vi "EminemExecuteLogic.vi"(9 "Feed_Vel_RPM":dbl, 10 "Shooter_Bottom_Vel_RPM":dbl, 11 "Shooter_Top_Vel_RPM":dbl) -> (0 "Box states":T1=enum."13-AmpDone", 1 "Shooter_Feed_Motor_Out":dbl, 2 "Shooter_Bottom_Motor_Out":dbl, 3 "Shooter_Top_Motor_Out":dbl)   [LabVIEW 2023]
uses:
  EminemStatesEnum.ctl
  <vilib>/Rock Robotics/WPI/ThirdParty/JAS_Junk/TrajLib/TypeDef/PID_ERROR_TOLERANCE.ctl
  <vilib>/Rock Robotics/WPI/ThirdParty/JAS_Junk/TrajLib/LinearFilter_ResetToValue.vi
  <vilib>/Rock Robotics/WPI/ThirdParty/JAS_Junk/TrajLib/LinearFilter_Calculate.vi
  <vilib>/Rock Robotics/WPI/ThirdParty/JAS_Junk/TrajLib/VI/BoolCmd_Recv_Internal.vi
  <vilib>/Rock Robotics/WPI/ThirdParty/JAS_Junk/TrajLib/Timer_New.vi
  Intake/IntakeGetHaveNote.vi
  <vilib>/Rock Robotics/WPI/ThirdParty/JAS_Junk/TrajLib/SlewRateLimiter_New.vi
  <vilib>/Rock Robotics/WPI/ThirdParty/JAS_Junk/TrajLib/SlewRateLimiter_Reset.vi
  <vilib>/Rock Robotics/WPI/ThirdParty/JAS_Junk/TrajLib/SlewRateLimiter_Calculate.vi
  <vilib>/Rock Robotics/WPI/ThirdParty/JAS_Junk/TrajLib/SlewRateLimiter_SetRate.vi
  <vilib>/Rock Robotics/WPI/ThirdParty/JAS_Junk/TrajLib/SimpleMotorFF_Calculate.vi
  <vilib>/Rock Robotics/WPI/ThirdParty/JAS_Junk/TrajLib/PIDController_AtSetpoint.vi
  <vilib>/Rock Robotics/WPI/ThirdParty/JAS_Junk/TrajLib/PIDController_SetPIDF.vi
  <vilib>/Rock Robotics/WPI/ThirdParty/JAS_Junk/TrajLib/PIDController_SetDerivativeFilter.vi
  <vilib>/Rock Robotics/WPI/ThirdParty/JAS_Junk/TrajLib/PIDController_SetIntegratorRange.vi
  <vilib>/Rock Robotics/WPI/ThirdParty/JAS_Junk/TrajLib/PIDController_SetTolerancePandV.vi
  <vilib>/Rock Robotics/WPI/ThirdParty/JAS_Junk/TrajLib/PIDController_DisableContinousInput.vi
  <vilib>/Rock Robotics/WPI/ThirdParty/JAS_Junk/TrajLib/PIDController_EnableContinousInput.vi
  <vilib>/Rock Robotics/WPI/ThirdParty/JAS_Junk/TrajLib/PIDController_Reset.vi
  <vilib>/Rock Robotics/WPI/ThirdParty/JAS_Junk/TrajLib/PIDController_New.vi
  <vilib>/Rock Robotics/WPI/ThirdParty/JAS_Junk/TrajLib/PIDController_SetOutputLimits.vi
  <vilib>/Rock Robotics/WPI/ThirdParty/JAS_Junk/TrajLib/VI/PIDController_SetIntegratorZone.vi
  <vilib>/Rock Robotics/WPI/ThirdParty/JAS_Junk/TrajLib/VI/BoolCmd_ObtainQueue.vi
  <vilib>/Rock Robotics/WPI/ThirdParty/JAS_Junk/TrajLib/Util_GetTime.vi
  <vilib>/Rock Robotics/WPI/ThirdParty/JAS_Junk/TrajLib/PIDController_NewPeriod.vi
  <vilib>/Rock Robotics/WPI/ThirdParty/JAS_Junk/TrajLib/VI/Util_GetTime_U32.vi
  <vilib>/Rock Robotics/SystemInterfaces/NetworkCommunication/NetComm_UsageReport_report.vi
  EminemGlobals.vi
  <vilib>/Utility/semaphor.llb/Obtain Semaphore Reference.vi
  <vilib>/Rock Robotics/WPI/ThirdParty/JAS_Junk/TrajLib/Timer_Reset.vi
  Intake/IntakeGlobal.vi
  Intake/IntakeCmdCancelALWAYS.vi
  <vilib>/Rock Robotics/WPI/ThirdParty/JAS_Junk/TrajLib/VI/Timer_Restart.vi
  <vilib>/Rock Robotics/WPI/ThirdParty/JAS_Junk/TrajLib/Timer_HasPeriodPassedOnce.vi
  Intake/IntakeCmdFeedToShootALWAYS.vi
  <vilib>/Rock Robotics/WPI/ThirdParty/JAS_Junk/TrajLib/VI/Util_GetTime_U64.vi
  <vilib>/Rock Robotics/WPI/ThirdParty/JAS_Junk/TrajLib/LinearFilter_MovingAverage.vi
  <vilib>/Rock Robotics/WPI/ThirdParty/JAS_Junk/TrajLib/LinearFilter_LowPassBW1.vi
  <vilib>/Rock Robotics/WPI/ThirdParty/JAS_Junk/TrajLib/LinearFilter_LowPassBW2.vi
  <vilib>/Rock Robotics/WPI/ThirdParty/JAS_Junk/TrajLib/LinearFilter_HighPassBW1.vi
  <vilib>/Rock Robotics/WPI/ThirdParty/JAS_Junk/TrajLib/LinearFilter_HighPassBW2.vi
  <vilib>/Rock Robotics/WPI/ThirdParty/JAS_Junk/TrajLib/Globals/Util_LibraryGlobals.vi
  <vilib>/Rock Robotics/WPI/ThirdParty/JAS_Junk/TrajLib/PIDController_AdvCalculate_FF_Sp_Pv.vi
  <vilib>/Rock Robotics/WPI/ThirdParty/JAS_Junk/TrajLib/Trajectory_Library.lvlib
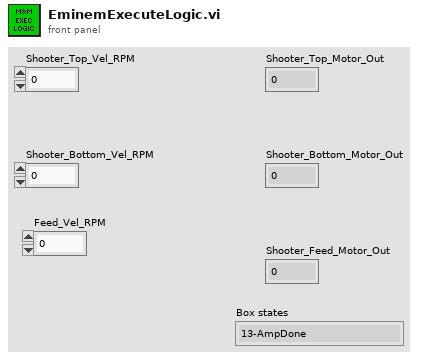
[diagram p1: front panel]
types:
  T1 = typedef "EminemStatesEnum.ctl" = enum16{"0-Init", "1-WaitForCmd", "2-Cancel", "3-ShootStart", "4-ShootRev", "5-RevUpStart", "6-ShootStartFeed&Timer", "7-ShootTimerOrSensorDone", "8-ShootDone", "9-AmpStart", "10-AmpUpToSpd?", "11-AmpStartFeed&Timer", "12-AmpTimerOrSensorDone", "13-AmpDone", "14-RevUpGetCmd"}
  T2 = enum16{"Moving Average", "Low Pass 1st Order Butterworth", "Low Pass 2nd Order Butterworth", "High Pass 1st Order Butterworth", "High Pass 2nd Order Butterworth"}
  T3 = typedef "Trajectory_Library.lvlib/PID_ERROR_TOLERANCE.ctl" = cluster{"PositionTolerance":dbl, "VelocityTolerance":dbl}
  T4 = typedef "Trajectory_Library.lvlib/SIMPLE_MOTOR_FF.ctl" = cluster{"Ks":dbl, "Kv":dbl, "Ka":dbl, "KnInv":dbl}
  T5 = typedef "Trajectory_Library.lvlib/PID_ADV_TUNING.ctl" = cluster{"Kf":dbl, "Kp":dbl, "Ki":dbl, "Kd":dbl, "MaximumIntegral":dbl, "MinimumIntegral":dbl, "Filter Derivative":bool, "IntegralZone":dbl}
  T6 = typedef "Trajectory_Library.lvlib/PID_ADV_LIMITS.ctl" = cluster{"MaxInput":dbl, "MinInput":dbl, "Continuous":bool, "MaxOutput":dbl, "MinOutput":dbl}
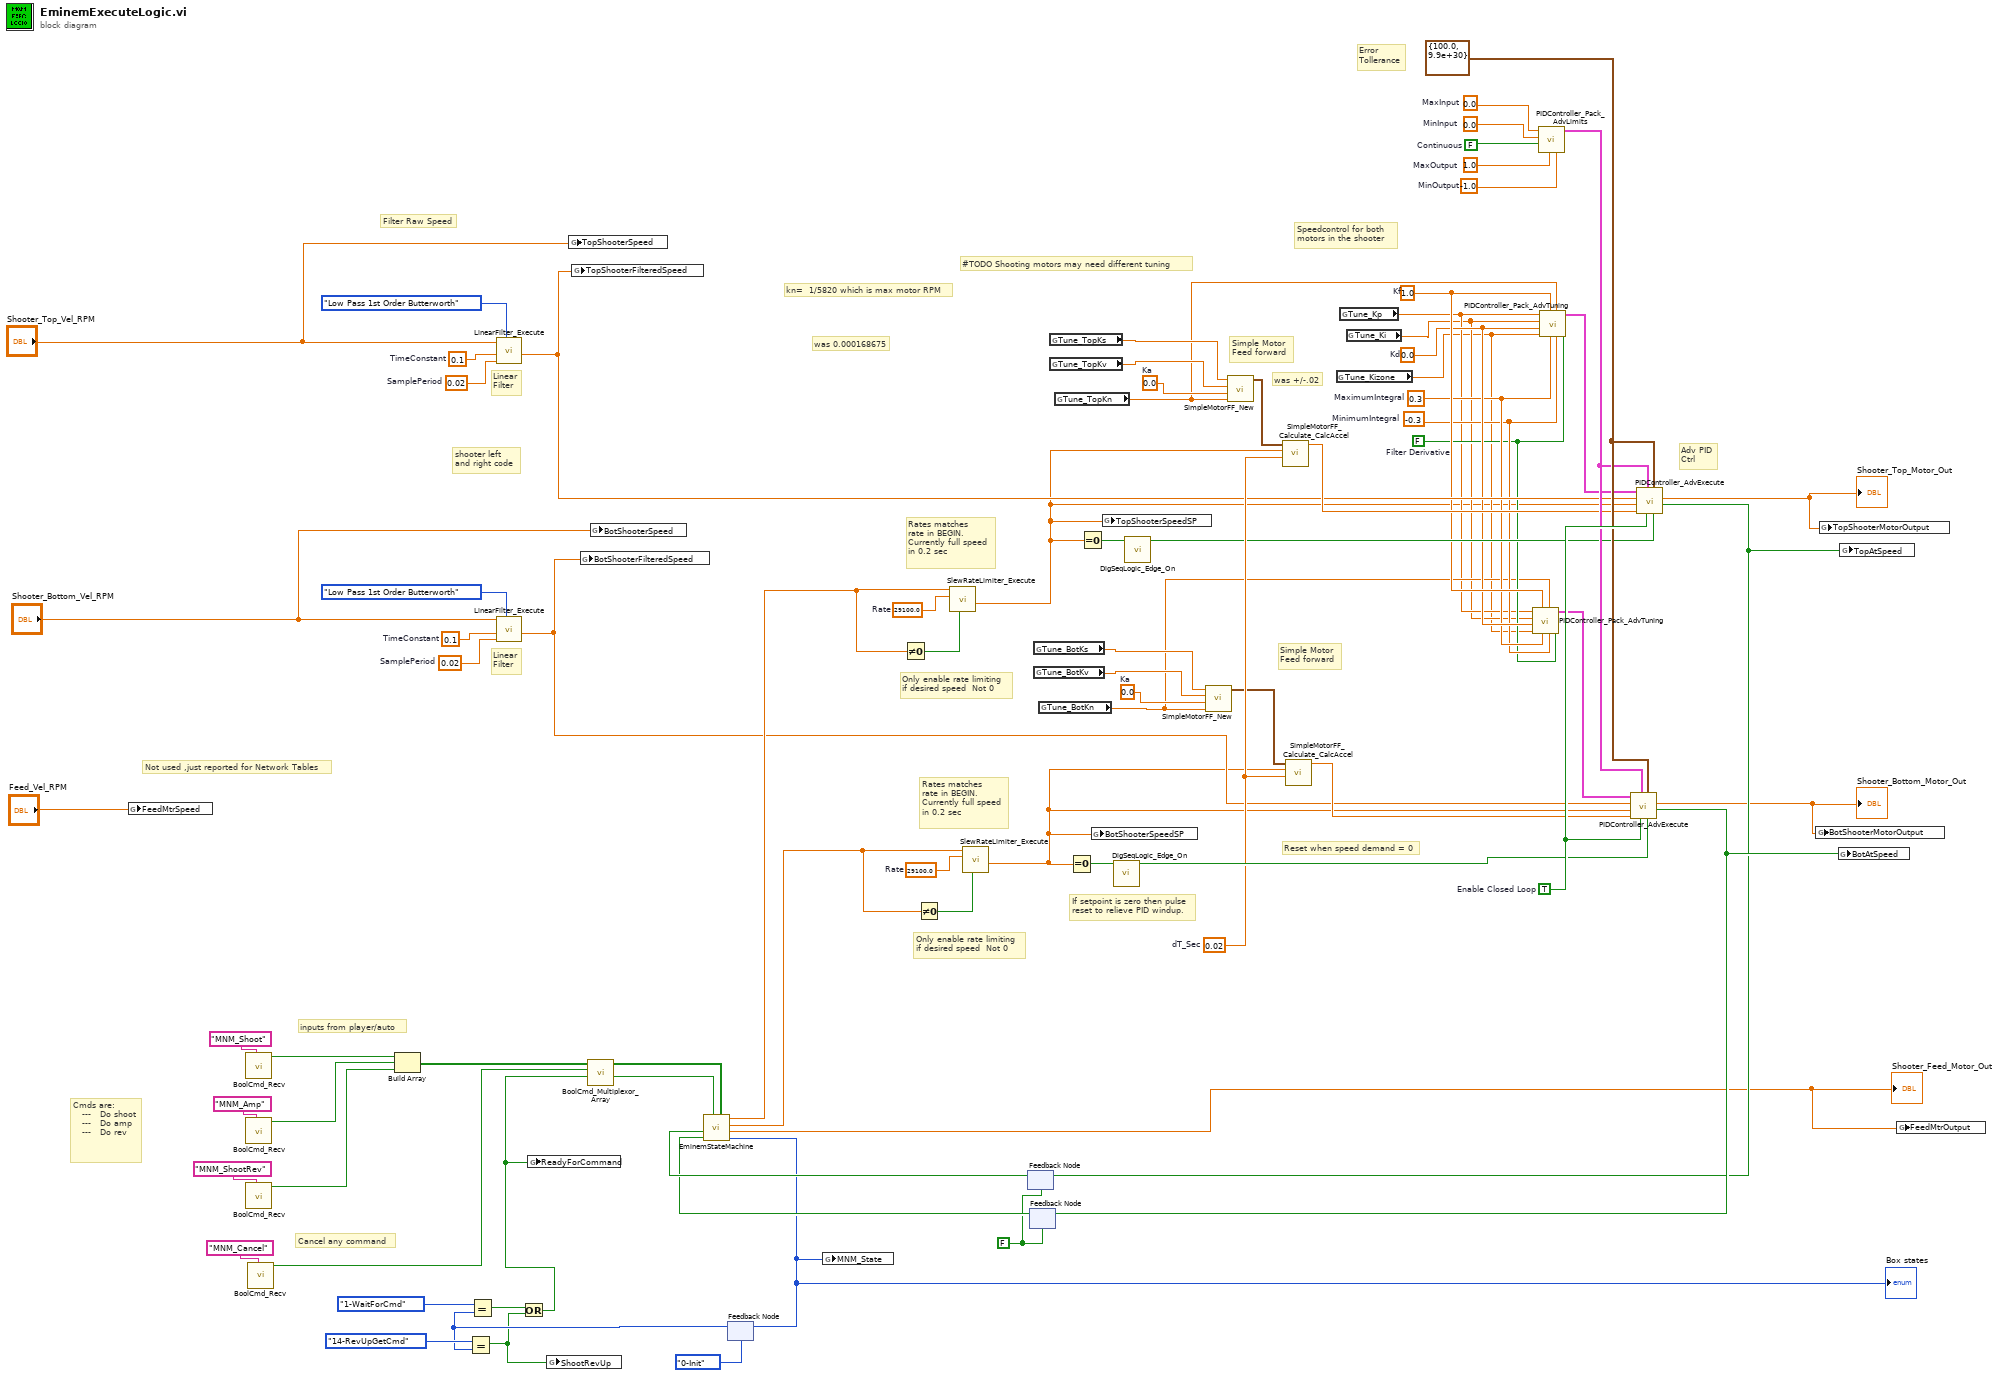
[diagram p0: block diagram]
diagram:
  w19 = 0.0  # Ka
  w26 = FALSE ("AtSetpoint")
  w42 = 29100.0  # Rate
  w79 = 29100.0  # Rate
  w74 = 0.02  # SamplePeriod
  w75 = 0.1  # TimeConstant
  w71 = 0.02  # SamplePeriod
  w72 = 0.1  # TimeConstant
  w81 = TRUE  # Enable Closed Loop
  w69 = T3 {"PositionTolerance"=100.0, "VelocityTolerance"=9.9e+30} ("PID Error Tolerance")
  w64 = 0.0  # Ka
  w15 = 0.0  # Kd
  w16 = 1.0  # Kf
  w14 = 0.3  # MaximumIntegral
  w13 = -0.3  # MinimumIntegral
  w12 = FALSE  # Filter Derivative
  w60 = 0.0  # MinInput
  w61 = FALSE  # Continuous
  w62 = 1.0  # MaxOutput
  w63 = -1.0  # MinOutput
  w59 = 0.0  # MaxInput
  w65 = 0.02  # dT_Sec
  # "Simple Motor\nFeed forward"
  # "was 0.000168675"
  # "#TODO Shooting motors may need different tuning"
  # "Not used ,just reported for Network Tables"
  # "Cmds are:\n   ---   Do shoot\n   ---   Do amp\n   ---   Do rev"
  # "Error \nTollerance"
  # "Filter Raw Speed"
  # "Rates matches\nrate in BEGIN.  \nCurrently full speed\nin 0.2 sec"
  # "Only enable rate limiting\nif desired speed  Not 0"
  # "Reset when speed demand = 0"
  # "was +/-.02"
  # "If setpoint is zero then pulse\nreset to relieve PID windup."
  # "Rates matches\nrate in BEGIN.  \nCurrently full speed\nin 0.2 sec"
  # "Only enable rate limiting\nif desired speed  Not 0"
  # "inputs from player/auto"
  # "Linear\nFilter"
  # "Linear\nFilter"
  # "Speedcontrol for both \nmotors in the shooter"
  # "Simple Motor\nFeed forward"
  # "Adv PID\nCtrl"
  # "Cancel any command"
  # "kn=  1/5820 which is max motor RPM"
  # "shooter left \nand right code"
  n1 = global write "EminemGlobals.vi" "FeedMtrSpeed"("Feed_Vel_RPM") -> ()
  n2 = call <vilib>:"BoolCmd_Recv.vi"("Command Name"="MNM_Shoot") -> ("New Request"=w52:bool)  [unwired: 9 in, 1 out]
  n3 = call <vilib>:"BoolCmd_Recv.vi"("Command Name"="MNM_Amp") -> ("New Request"=w51:bool)  [unwired: 9 in, 1 out]
  n4 = call <vilib>:"BoolCmd_Recv.vi"("Command Name"="MNM_ShootRev") -> ("New Request"=w49:bool)  [unwired: 9 in, 1 out]
  n5 = call <vilib>:"BoolCmd_Recv.vi"("Command Name"="MNM_Cancel") -> ("New Request"=w54:bool)  [unwired: 9 in, 1 out]
  n6 = Build Array(w52, w51, w49) -> (w53:bool[])
  n7 = call <vilib>:"LinearFilter_Execute.vi"("Filter Type"=T2."Low Pass 1st Order Butterworth", "SamplePeriod"=w74, "TimeConstant"=w75, "Input"="Shooter_Top_Vel_RPM") -> ("Output"=w28:dbl)  [unwired: 6 in, 1 out]
  n8 = call <vilib>:"LinearFilter_Execute.vi"("Filter Type"=T2."Low Pass 1st Order Butterworth", "SamplePeriod"=w71, "TimeConstant"=w72, "Input"="Shooter_Bottom_Vel_RPM") -> ("Output"=w30:dbl)  [unwired: 6 in, 1 out]
  n9 = global write "EminemGlobals.vi" "TopShooterSpeed"("Shooter_Top_Vel_RPM") -> ()
  n10 = global write "EminemGlobals.vi" "TopShooterFilteredSpeed"(w28) -> ()
  n11 = global write "EminemGlobals.vi" "BotShooterFilteredSpeed"(w30) -> ()
  n12 = global write "EminemGlobals.vi" "BotShooterSpeed"("Shooter_Bottom_Vel_RPM") -> ()
  n13 = feedback #1(EminemStatesEnum."0-Init" ("Box states")) -> (w23:T1)
  n14 = Equal?(x=EminemStatesEnum."14-RevUpGetCmd" ("Box states"), y=w23) -> (x = y?=w20:bool)
  n15 = Equal?(x=EminemStatesEnum."1-WaitForCmd" ("Box states"), y=w23) -> (x = y?=w22:bool)
  n16 = Or(x=w22, y=w20) -> (x .or. y?=w21:bool)
  n17 = global write "EminemGlobals.vi" "ReadyForCommand"(w21) -> ()
  n18 = global write "EminemGlobals.vi" "ShootRevUp"(w20) -> ()
  n19 = call <vilib>:"BoolCmd_Multiplexor_Array.vi"("Ready"=w21, "Command Cancel"=w54, "Commands"=w53) -> ("Do Cancel"=w45:bool, "Do Command"=w46:bool[])  [unwired: 7 in]
  n20 = feedback #2(w26) -> (w41:bool)
  n21 = feedback #3(w26) -> (w40:bool)
  n22 = call "EminemStateMachine.vi"("EminemCommand"=w46, "EminemCancel"=w45, "LowerShoot_At_Speed"=w40, "UpperShoot_At_Speed"=w41) -> ("Box states"=w37:T1, "AmpAndFeed-MotorDmd"=w32:dbl, "LowerShooter-RPM_Dmd"=w39:dbl, "UpperShooterAndAmp-RPM_Dmd"=w38:dbl)  [unwired: 4 in]
  "Shooter_Feed_Motor_Out" <- w32
  "Box states" <- w37
  n23 = feedback-in #1(w37) -> ()
  n24 = global write "EminemGlobals.vi" "MNM_State"(w37) -> ()
  n25 = Not Equal To 0?(x=w38) -> (x != 0?=w43:bool)
  n26 = Not Equal To 0?(x=w39) -> (x != 0?=w80:bool)
  n27 = call <vilib>:"SlewRateLimiter_Execute.vi"("Enable"=w43, "PositiveRate"=w42, "Input"=w38) -> ("Output"=w2:dbl)  [unwired: 7 in, 1 out]
  n28 = call <vilib>:"SlewRateLimiter_Execute.vi"("Enable"=w80, "PositiveRate"=w79, "Input"=w39) -> ("Output"=w1:dbl)  [unwired: 7 in, 1 out]
  n29 = global read "EminemGlobals.vi" "Tune_BotKs"() -> (w8:dbl)
  n30 = global read "EminemGlobals.vi" "Tune_BotKv"() -> (w7:dbl)
  n31 = global read "EminemGlobals.vi" "Tune_BotKn"() -> (w6:dbl)
  n32 = global read "EminemGlobals.vi" "Tune_TopKs"() -> (w11:dbl)
  n33 = global read "EminemGlobals.vi" "Tune_TopKv"() -> (w10:dbl)
  n34 = global read "EminemGlobals.vi" "Tune_TopKn"() -> (w9:dbl)
  n35 = Equal To 0?(x=w1) -> (x = 0?=w77:bool)
  n36 = Equal To 0?(x=w2) -> (x = 0?=w48:bool)
  n37 = global write "EminemGlobals.vi" "BotShooterSpeedSP"(w1) -> ()
  n38 = global write "EminemGlobals.vi" "TopShooterSpeedSP"(w2) -> ()
  n39 = call <vilib>:"DigSeqLogic_Edge_On.vi"("Input"=w77) -> ("On Edge"=w78:bool)  [unwired: 10 in]
  n40 = call <vilib>:"DigSeqLogic_Edge_On.vi"("Input"=w48) -> ("On Edge"=w47:bool)  [unwired: 10 in]
  n41 = call <vilib>:"SimpleMotorFF_New.vi"("Kn"=w6, "Ka"=w19, "Kv"=w7, "Ks"=w8) -> ("SIMPLE_MOTOR_FF"=w18:T4)  [unwired: 7 in]
  n42 = call <vilib>:"SimpleMotorFF_New.vi"("Kn"=w9, "Ka"=w64, "Kv"=w10, "Ks"=w11) -> ("SIMPLE_MOTOR_FF"=w66:T4)  [unwired: 7 in]
  n43 = call <vilib>:"SimpleMotorFF_Calculate_CalcAccel.vi"("dT_Sec"=w65, "VelSp"=w2, "SIMPLE_MOTOR_FF"=w66) -> ("FeedForward"=w58:dbl)  [unwired: 8 in]
  n44 = call <vilib>:"SimpleMotorFF_Calculate_CalcAccel.vi"("dT_Sec"=w65, "VelSp"=w1, "SIMPLE_MOTOR_FF"=w18) -> ("FeedForward"=w70:dbl)  [unwired: 8 in]
  n45 = global read "EminemGlobals.vi" "Tune_Kizone"() -> (w3:dbl)
  n46 = global read "EminemGlobals.vi" "Tune_Kp"() -> (w5:dbl)
  n47 = global read "EminemGlobals.vi" "Tune_Ki"() -> (w4:dbl)
  n48 = call <vilib>:"PIDController_Pack_AdvTuning.vi"("Filter Derivative"=w12, "MinimumIntegral"=w13, "Kn"=w6, "MaximumIntegral"=w14, "Kf"=w16, "IntegralZone"=w3, "Kd"=w15, "Ki"=w4, "Kp"=w5) -> ("Adv PID Tuning"=w17:T5)  [unwired: 2 in]
  n49 = call <vilib>:"PIDController_Pack_AdvLimits.vi"("MinOutput"=w63, "MaxOutput"=w62, "Continuous"=w61, "MinInput"=w60, "MaxInput"=w59) -> ("Adv PID Limits"=w68:T6)  [unwired: 6 in]
  n50 = call <vilib>:"PIDController_Pack_AdvTuning.vi"("Filter Derivative"=w12, "MinimumIntegral"=w13, "Kn"=w9, "MaximumIntegral"=w14, "Kf"=w16, "IntegralZone"=w3, "Kd"=w15, "Ki"=w4, "Kp"=w5) -> ("Adv PID Tuning"=w67:T5)  [unwired: 2 in]
  n51 = call <vilib>:"PIDController_AdvExecute.vi"("Reset"=w78, "PID Error Tolerance"=w69, "Auto"=w81, "Adv PID Limits"=w68, "FF-FeedForward"=w70, "SP-SetPoint"=w1, "PV-Measurement"=w30, "Adv PID Tuning"=w17) -> ("AtSetpoint"=w36:bool, "CO-ControlOutput"=w33:dbl)  [unwired: 1 in, 1 out]
  "Shooter_Bottom_Motor_Out" <- w33
  n52 = feedback-in #3(w36) -> ()
  n53 = call <vilib>:"PIDController_AdvExecute.vi"("Reset"=w47, "PID Error Tolerance"=w69, "Auto"=w81, "Adv PID Limits"=w68, "FF-FeedForward"=w58, "SP-SetPoint"=w2, "PV-Measurement"=w28, "Adv PID Tuning"=w67) -> ("AtSetpoint"=w35:bool, "CO-ControlOutput"=w34:dbl)  [unwired: 1 in, 1 out]
  "Shooter_Top_Motor_Out" <- w34
  n54 = feedback-in #2(w35) -> ()
  n55 = global write "EminemGlobals.vi" "BotShooterMotorOutput"(w33) -> ()
  n56 = global write "EminemGlobals.vi" "TopShooterMotorOutput"(w34) -> ()
  n57 = global write "EminemGlobals.vi" "BotAtSpeed"(w36) -> ()
  n58 = global write "EminemGlobals.vi" "TopAtSpeed"(w35) -> ()
  n59 = global write "EminemGlobals.vi" "FeedMtrOutput"(w32) -> ()
